vi "20150714분석기.vi"() -> ()   [LabVIEW 2014]
uses:
  <vilib>/Utility/file.llb/Read From Spreadsheet File (string).vi
panel:
  out "경로 7":path
  out "경로 6":path
  out "경로 5":path
  out "경로 4":path
  out "경로 3":path
  out "경로 2":path
  out "경로":path
  in  "Name":path
  in  "Save_path":path
  in  "Online_Path":path
  in  "Training_Path":path
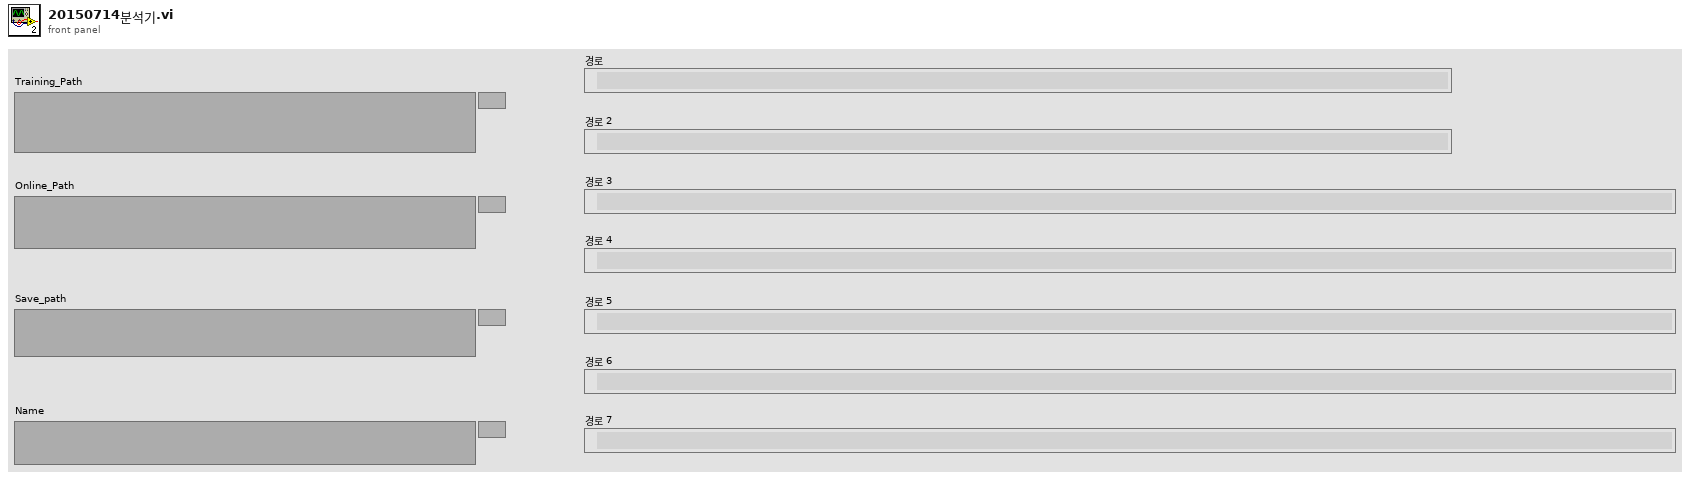
[diagram p1: front panel]
diagram:
  n1 = call-poly <vilib>:"Read From Spreadsheet File.vi"("transpose (no:F)"=TRUE, "file path (dialog if empty)"="Training_Path") -> ("first row"=w10:string[])  [unwired: 5 in, 4 out]
  n2 = call-poly <vilib>:"Read From Spreadsheet File.vi"("transpose (no:F)"=TRUE, "file path (dialog if empty)"="Online_Path") -> ("first row"=w7:string[])  [unwired: 5 in, 4 out]
  n3 = call-poly <vilib>:"Read From Spreadsheet File.vi"("transpose (no:F)"=TRUE, "file path (dialog if empty)"="Save_path") -> ("first row"=w4:string[])  [unwired: 5 in, 4 out]
  n4 = call-poly <vilib>:"Read From Spreadsheet File.vi"("transpose (no:F)"=TRUE, "file path (dialog if empty)"="Name") -> ("first row"=w1:string[])  [unwired: 5 in, 4 out]
  n5 = for {
    tunnel: w10 -> [w14] mode=indexing
    tunnel: w7 -> [w13] mode=indexing
    tunnel: w4 -> [w25] mode=indexing
    tunnel: w1 -> [w15] mode=indexing
    # "1) Training_Path.txt\n2) Online_Path.txt\n3) Save_Path.txt\n4) Name.txt\n를 저장한\ntxt파일을 불러온후 실행하시면 됩니다."
    n6 = Concatenate Strings(w14, "\\ERP_Parameters_of_Target_prior.txt" ("string")) -> (w19:string)
    n7 = Concatenate Strings(w14, "\\ERP_Parameters_of_NonTarget_prior.txt" ("string")) -> (w18:string)
    n8 = String To Path(string=w19) -> (path=w17:path)
    "경로" <- w17
    n9 = String To Path(string=w18) -> (path=w16:path)
    "경로 2" <- w16
    n10 = flat-sequence {
      tunnel: [w61] -> w40
      tunnel: [w60] -> w39
      tunnel: [w43] -> w38
      tunnel: [w42] -> w37
      tunnel: [w41] -> w36
      tunnel: [w59] -> w22
      tunnel: w13 -> [w45]
      tunnel: w14 -> [w60]
      tunnel: w25 -> [w59]
      tunnel: w15 -> [w61]
      tunnel: w40 -> [w68]
      tunnel: [w68] -> w35
      tunnel: w39 -> [w70]
      tunnel: [w70] -> w34
      tunnel: w38 -> [w71]
      tunnel: [w71] -> w33
      tunnel: w37 -> [w63]
      tunnel: [w63] -> w32
      tunnel: w36 -> [w62]
      tunnel: [w62] -> w31
      tunnel: [w66] -> w23
      tunnel: w22 -> [w66]
      tunnel: w17 -> [w65]
      tunnel: w16 -> [w64]
      tunnel: [w87] -> w30
      tunnel: [w85] -> w29
      tunnel: [w92] -> w28
      tunnel: [w91] -> w27
      tunnel: [w90] -> w26
      tunnel: [w89] -> w24
      tunnel: w23 -> [w89]
      tunnel: w31 -> [w90]
      tunnel: w32 -> [w91]
      tunnel: w33 -> [w92]
      tunnel: w34 -> [w85]
      tunnel: w35 -> [w87]
      tunnel: w24 -> [w106]
      tunnel: w26 -> [w109]
      tunnel: w27 -> [w107]
      tunnel: w28 -> [w110]
      tunnel: w29 -> [w105]
      tunnel: w30 -> [w108]
      tunnel: w16 -> [w114]
      tunnel: w17 -> [w113]
      frame #0 {
        # "FLDA"
        n11 = Concatenate Strings(w61, "_FLDA" ("string")) -> (w57:string)
        n12 = Concatenate Strings(w60, "\\LDA_Matrix_Value_prior.txt" ("string")) -> (w48:string)
        n13 = Concatenate Strings(w60, "\\Weight_Vector_prior.txt" ("string")) -> (w47:string)
        n14 = Concatenate Strings(w45, "\\Target_order.txt" ("string")) -> (w53:string)
        n15 = Concatenate Strings(w45, "\\mius_flash_order.txt" ("string")) -> (w52:string)
        n16 = Concatenate Strings(w45, "\\Brain.txt" ("string")) -> (w51:string)
        n17 = String To Path(string=w48) -> (path=w46:path)
        "경로 3" <- w46
        n18 = String To Path(string=w47) -> (path=w44:path)
        "경로 4" <- w44
        n19 = String To Path(string=w52) -> (path=w42:path)
        "경로 6" <- w42
        n20 = String To Path(string=w51) -> (path=w41:path)
        "경로 7" <- w41
        n21 = String To Path(string=w53) -> (path=w43:path)
        "경로 5" <- w43
        n22 = call "Offline_Analysis_FLDA_분석기.vi"("LDA_matrix"=w46, "Weight"=w44, "Target_order.txt"=w43, "mius_flash_order"=w42, "Brain"=w41, "피험자이름"=w57, "Save_path"=w59) -> ()  [unwired: 9 in]
      }
      frame #1 {
        # "SVM"
        n23 = Concatenate Strings(w68, "_SVM" ("string")) -> (w67:string)
        n24 = disable-structure shown="비활성화" {
          disable-tunnel: w71 -> [w84 _]
          disable-tunnel: w70 -> [w83 _]
          disable-tunnel: w67 -> [w82 _]
          disable-tunnel: w66 -> [w80 _]
          disable-tunnel: w65 -> [w79 _]
          disable-tunnel: w64 -> [w78 _]
          disable-tunnel: w63 -> [w75 _]
          disable-tunnel: w62 -> [w74 _]
          frame Disabled {
            n25 = Concatenate Strings(w83, "\\LDA_Matrix_Value_SWLDA.txt" ("string")) -> (w77:string)
            n26 = Concatenate Strings(w83, "\\svm_model.model" ("string")) -> (w81:string)
            n27 = String To Path(string=w77) -> (path=w76:path)
            n28 = call "Offline_Analysis_SVM_분석기.vi"("LDA_matrix"=w76, "Target"=w79, "Nontarget"=w78, "Target_order.txt"=w84, "mius_flash_order"=w75, "Brain"=w74, "svm_model_file"=w81, "피험자이름"=w82, "Save_path"=w80) -> ()  [unwired: 7 in]
          }
          frame Enabled {
          }
        }
      }
      frame #2 {
        # "SWLDA (LDA)"
        n29 = Concatenate Strings(w87, "_SWLDA" ("string")) -> (w86:string)
        n30 = disable-structure shown="비활성화" {
          disable-tunnel: w92 -> [w104 _]
          disable-tunnel: w91 -> [w103 _]
          disable-tunnel: w90 -> [w102 _]
          disable-tunnel: w89 -> [w101 _]
          disable-tunnel: w86 -> [w94 _]
          disable-tunnel: w85 -> [w93 _]
          frame Disabled {
            # "p-enter = 0.01\np-remove = 0.05"
            n31 = Concatenate Strings(w93, "\\LDA_Matrix_Value_SWLDA.txt") -> (w98:string)
            n32 = Concatenate Strings(w93, "\\Weight_Vector_SWLDA.txt") -> (w97:string)
            n33 = String To Path(string=w98) -> (path=w96:path)
            n34 = String To Path(string=w97) -> (path=w95:path)
            n35 = call "Offline_Analysis__SWLDA_분석기.vi"("LDA_matrix"=w96, "Weight"=w95, "Target_order.txt"=w104, "mius_flash_order"=w103, "Brain"=w102, "피험자이름"=w94, "Save_path"=w101) -> ()  [unwired: 9 in]
          }
          frame Enabled {
          }
        }
      }
      frame #3 {
        # "p-enter = 0.01\np-remove = 0.05"
        # "SWSVM_New (in)"
        n36 = Concatenate Strings(w108, "_SWSVM" ("string")) -> (w112:string)
        n37 = disable-structure shown="비활성화" {
          disable-tunnel: w114 -> [w130 _]
          disable-tunnel: w113 -> [w129 _]
          disable-tunnel: w112 -> [w128 _]
          disable-tunnel: w110 -> [w127 _]
          disable-tunnel: w109 -> [w126 _]
          disable-tunnel: w107 -> [w125 _]
          disable-tunnel: w106 -> [w124 _]
          disable-tunnel: w105 -> [w115 _]
          frame Disabled {
            n38 = Concatenate Strings(w115, "\\svm_model2.model") -> (w120:string)
            n39 = Concatenate Strings(w115, "\\LDA_Matrix_Value_SWLDA.txt") -> (w118:string)
            n40 = Concatenate Strings(w115, "\\in_SWLDA.txt") -> (w119:string)
            n41 = String To Path(string=w118) -> (path=w122:path)
            n42 = String To Path(string=w119) -> (path=w117:path)
            n43 = call "Offline_Analysis_SWSVM_newSelectionMethod_in_분석기.vi"("LDA_matrix"=w122, "Target"=w129, "Nontarget"=w130, "in_matrix"=w117, "svm_model_file"=w120, "Target_order.txt"=w127, "mius_flash_order"=w125, "Brain"=w126, "피험자이름"=w128, "Save_path"=w124) -> ()  [unwired: 6 in]
          }
          frame Enabled {
          }
        }
      }
    }
  }
